vi "Update Addresses.vi"(8 "error in (no error)":errorcluster, 10 "Names":string[](array[string]), 11 "Chat Window Panel in":refnum<class "Chat Window Panel.lvclass">) -> (0 "error out":errorcluster, 3 "Chat Window Panel out":refnum<class "Chat Window Panel.lvclass">)   [LabVIEW 2018, in "Chat Window Panel.lvlib" / "Chat Window Panel.lvclass"]
uses:
  Chat Window Panel.lvclass
  Chat Window Panel.lvclass/Chat Window Panel.ctl
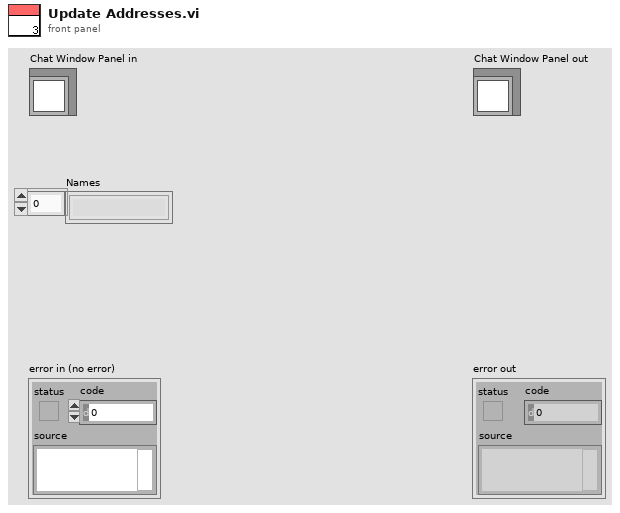
[diagram p1: front panel]
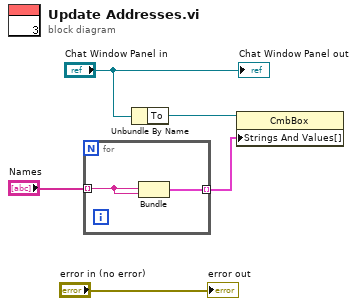
[diagram p0: block diagram]
diagram:
  n1 = for {
    tunnel: "Names" -> [w7] mode=indexing
    tunnel: [w6] -> w1 mode=indexing
    n2 = Bundle("String"=w7, "String"=w7) -> (w6:cluster{"String":string, "String":string})  [unwired: 1 in]
  }
  n3 = Unbundle By Name("Chat Window Panel in") -> ("To"=w4:refnum<vi>)
  n4 = property class="CmbBox"(reference=w4, "Strings And Values[]"=w1) -> ()  [unwired: 1 in, 2 out]
  "error out" <- "error in (no error)"
  "Chat Window Panel out" <- "Chat Window Panel in"
